vi "Sequence Data 2d Array to Cluster.vi"(0 "data":string[][](array[string])) -> (5 "Array":T1[](array[typedef]), 6 "Variance":string[](array[string]), 7 "Test System":string[](array[string]), 8 "Chart Scale":string[](array[string]), 9 "Test Media":string[](array[string]), 10 "Cycle":string[](array[string]))   [LabVIEW 2020]
uses:
  Control/Setup - Single Sequence.ctl
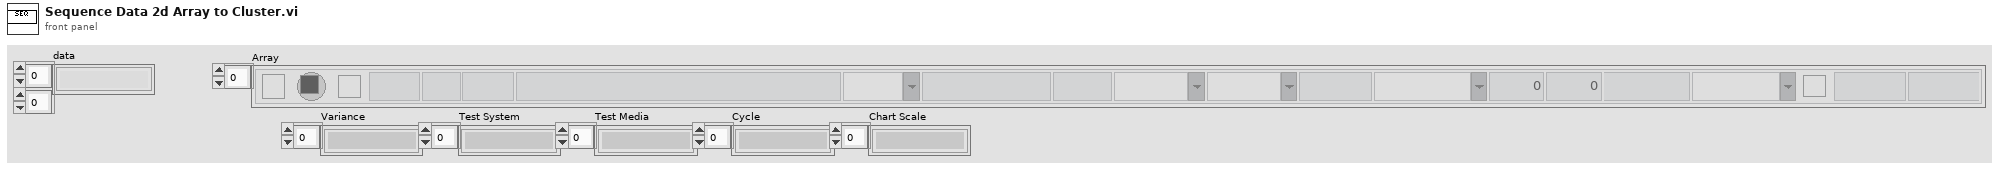
[diagram p1: front panel]
types:
  T1 = typedef "Setup - Single Sequence.ctl" = cluster{"Seq.Select":bool, "Seq.Status":u32, "Seq.Run":bool, "Seq.TestSequence":string, "Seq.No":string, "Seq.TestReq":string, "Seq.TestProcedure":string, "Seq.Section":string, "Seq.TestPressure":string, "Seq.TestGroup":string, "Seq.MSHP":dbl, "Seq.PHPD":dbl, "Seq.HoldingTime":string, "Seq.ChartScale":string, "Seq.ActuatorPressure":string, "Seq.MaxBDPressure":string, "Seq.BDIndicator":bool, "Seq.TestMedia":string, "Seq.Variance":string, "Seq.TestCycle":string, "Seq.TestSystem":string}
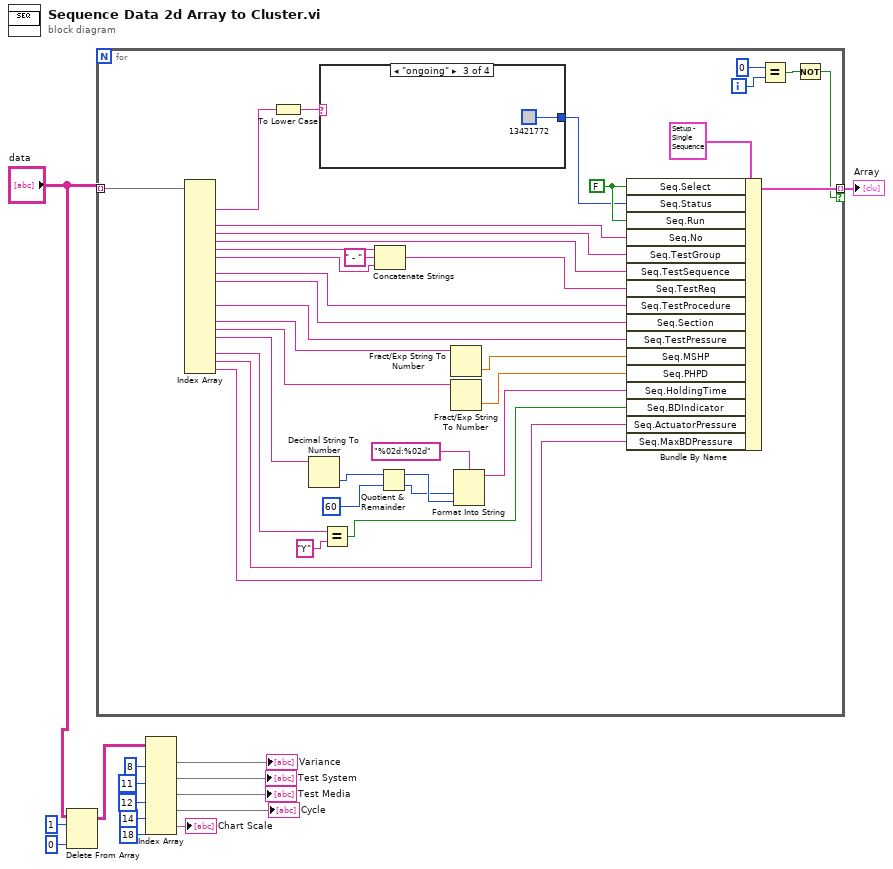
[diagram p0: block diagram]
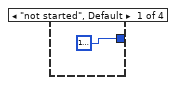
[diagram p2: hidden frame]
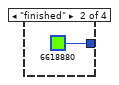
[diagram p3: hidden frame]
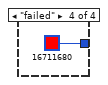
[diagram p4: hidden frame]
diagram:
  n1 = Delete From Array(array="data", length=1, index (col)=0 ("disabled index (col)")) -> (array with subset deleted=w7:string[][])  [unwired: 1 in, 1 out]
  n2 = for {
    tunnel: "data" -> [w19] mode=indexing
    tunnel: [w52] -> w15 mode=indexing if=w48
    i -> [w51]
    w40 = FALSE ("Seq.Select")
    n3 = Index Array(array=w19) -> (element #2=w38:string, element #4=w37:string, element #5=w36:string, element #6=w35:string, element #7=w34:string, element #8=w32:string, element #10=w30:string, element #11=w29:string, element #14=w26:string, element #16=w25:string, element #17=w24:string, element #18=w23:string, element #20=w16:string, element #21=w17:string, element #22=w18:string)  [unwired: 22 in, 7 out]
    n4 = To Lower Case(string=w38) -> (all lower case string=w42:string)
    n5 = Decimal String To Number(string=w23) -> (number=w47:i32)  [unwired: 2 in, 1 out]
    n6 = case shown="\"ongoing\"" w42 {
      tunnel: [u32 16777226 u32 6618880 u32 13421772 u32 16711680] -> w39
      frame "not started", Default {
      }
      frame "finished" {
      }
      frame "ongoing" {
      }
      frame "failed" {
      }
    }
    n7 = Equal?(x=w16, y="Y" ("string")) -> (x = y?=w20:bool)
    n8 = Concatenate Strings(w34, " - " ("string"), w32) -> (w31:string)
    n9 = Quotient & Remainder(x=w47, y=60) -> (x-y*floor(x/y)=w45:i32, floor(x/y)=w44:i32)
    n10 = Fract/Exp String To Number(string=w25) -> (number=w28:dbl)  [unwired: 3 in, 1 out]
    n11 = Fract/Exp String To Number(string=w24) -> (number=w27:dbl)  [unwired: 3 in, 1 out]
    n12 = Format Into String(format string="%02d:%02d", w44, w45) -> (resulting string=w22:string)  [unwired: 2 in, 1 out]
    n13 = Bundle By Name(cluster=T1 {"Seq.Select"=FALSE, "Seq.Status"=16777215, "Seq.Run"=FALSE, "Seq.TestSequence"="", "Seq.No"="", "Seq.TestReq"="", "Seq.TestProcedure"="", "Seq.Section"="", "Seq.TestPressure"="", "Seq.TestGroup"="", "Seq.MSHP"=0.0, "Seq.PHPD"=0.0, "Seq.HoldingTime"="", "Seq.ChartScale"="", "Seq.ActuatorPressure"="", "Seq.MaxBDPressure"="", "Seq.BDIndicator"=FALSE, "Seq.TestMedia"="", "Seq.Variance"="", "Seq.TestCycle"="", "Seq.TestSystem"=""} ("Setup - Sequence Data"), "Seq.Select"=w40, "Seq.Status"=w39, "Seq.Run"=w40, "Seq.No"=w37, "Seq.TestGroup"=w36, "Seq.TestSequence"=w35, "Seq.TestReq"=w31, "Seq.TestProcedure"=w30, "Seq.Section"=w29, "Seq.TestPressure"=w26, "Seq.MSHP"=w28, "Seq.PHPD"=w27, "Seq.HoldingTime"=w22, "Seq.BDIndicator"=w20, "Seq.ActuatorPressure"=w17, "Seq.MaxBDPressure"=w18) -> (w52:T1)
    n14 = Equal?(x=0, y=w51) -> (x = y?=w49:bool)
    n15 = Not(x=w49) -> (.not. x?=w48:bool)
  }
  "Array" <- w15
  n16 = Index Array(array=w7, index (col) #1=8 ("disabled index (col)"), index (col) #2=11 ("index (col)"), index (col) #3=12 ("index (col)"), index (col) #4=14 ("index (col)"), index (col) #5=18 ("index (col)")) -> (element #1=→"Variance":string[], element #2=→"Test System":string[], element #3=→"Test Media":string[], element #4=→"Cycle":string[], element #5=→"Chart Scale":string[])  [unwired: 5 in]
